vi "Concatenate Non-Empty Strings.vi"(6 "String2":string, 8 "String1":string) -> (2 "Result String":string)   [LabVIEW 2017, in "CSM Shared.lvlib"]
uses:
  CSM Shared.lvlib
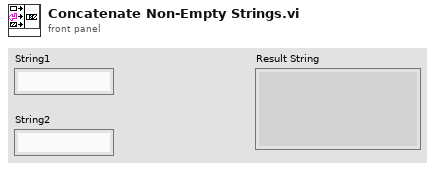
[diagram p1: front panel]
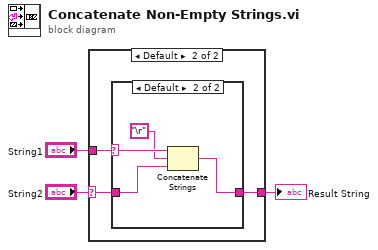
[diagram p0: block diagram]
diagram:
  n1 = case shown="Default" "String2" {
    selector: "String2" -> [_ w6]
    tunnel: [w4 w7] -> w1
    tunnel: "String1" -> [w4 w5]
    frame "" {
    }
    frame Default {
      n2 = case shown="Default" w5 {
        selector: w5 -> [_ w11]
        tunnel: [w8 w12] -> w7
        tunnel: w6 -> [w8 w9]
        frame "" {
        }
        frame Default {
          n3 = Concatenate Strings(w11, "\r", w9) -> (w12:string)
        }
      }
    }
  }
  "Result String" <- w1
